vi "Ack_estado_Arduino.vi"(8 "error in (no error)":errorcluster, 10 "Enum":T1, 11 "VISA resource name":refnum<visa-resource-name>) -> (0 "error out":errorcluster, 2 "read buffer":string, 3 "VISA resource name out":refnum<visa-resource-name>)   [LabVIEW 2019, in "SHARED VI'S.lvlib"]
uses:
  SHARED VI'S.lvlib
  LVPROJ_MOVIMIENTO_CABEZAL/LABVIEW_MOVIMIENTO/MOVIMIENTO CABEZAL/Typedefs/Estados_arduino.ctl
  <vilib>/Utility/error.llb/Error Cluster From Error Code.vi
  <vilib>/ErrorRing/Error Ring.xnode
panel:
  out "numero de datos leidos":u32
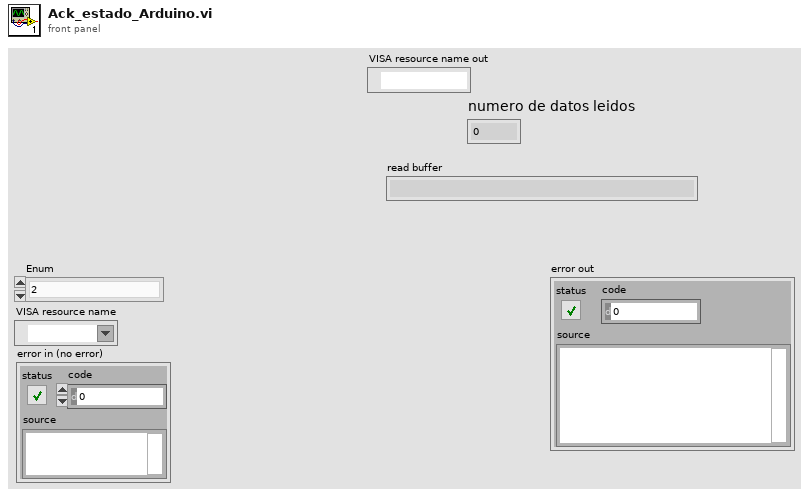
[diagram p1: front panel]
types:
  T1 = typedef "Estados_arduino.ctl" = enum16{"2", "3", "4", "5", "6", "7", "9", "8"}
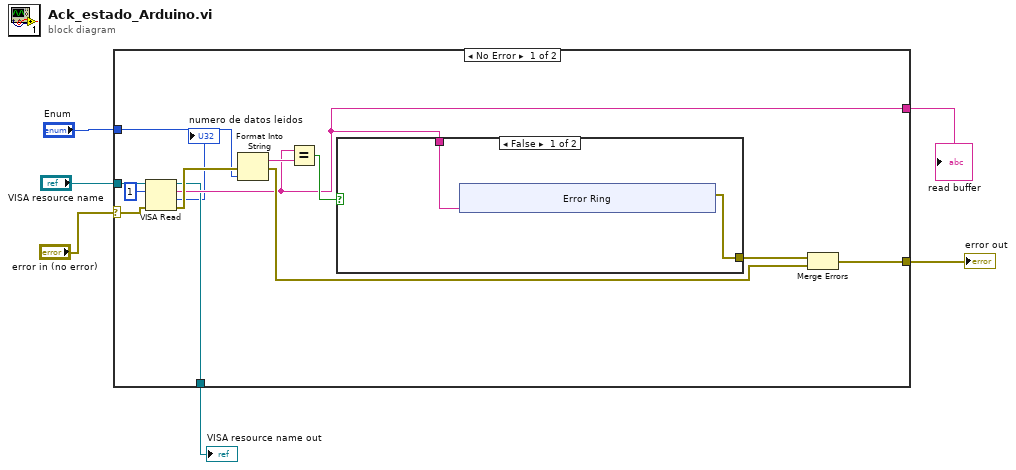
[diagram p0: block diagram]
diagram:
  n1 = case shown="No Error" "error in (no error)" {
    selector: "error in (no error)" -> [w11 w30]
    tunnel: "VISA resource name" -> [w19 w29]
    tunnel: [w14 _] -> w5
    tunnel: [w12 w30] -> w4
    tunnel: [w10 w29] -> w2
    tunnel: "Enum" -> [w9 _]
    frame No Error {
      n2 = VISA Read(VISA resource name=w19, byte count=u32 1, error in (no error)=w11) -> (VISA resource name out=w10:refnum<visa-resource-name>, read buffer=w14:string, return count=→"numero de datos leidos":u32, error out=w16:errorcluster)
      n3 = Format Into String(error in=w16, w9) -> (resulting string=w18:string, error out=w15:errorcluster)  [unwired: 2 in]
      n4 = Equal?(x=w14, y=w18) -> (x = y?=w17:bool)
      n5 = case shown="False" w17 {
        tunnel: w14 -> [w21 _]
        tunnel: [w20 _] -> w13
        frame False {
          n6 = xnode ("Error Ring")("parameter 0"=w21) -> ("error out"=w20:errorcluster)
        }
        frame True {
        }
      }
      n7 = Merge Errors(w13, w15) -> (w12:errorcluster)
    }
    frame Error {
    }
  }
  "error out" <- w4
  "VISA resource name out" <- w2
  "read buffer" <- w5
